vi "przygotowanie sygnalu do Mixed Graph.vi"() -> ()   [LabVIEW 2013]
uses:
  <vilib>/Waveform/DWDTOps.llb/DWDT Boolean Array to Digital.vi
panel:
  out "found":bool
  out "values":string
  out "transposed array":bool[][](array[boolean])
  in  "Array":bool[](array[boolean])
  out "Mixed Signal Graph":T1(graph)
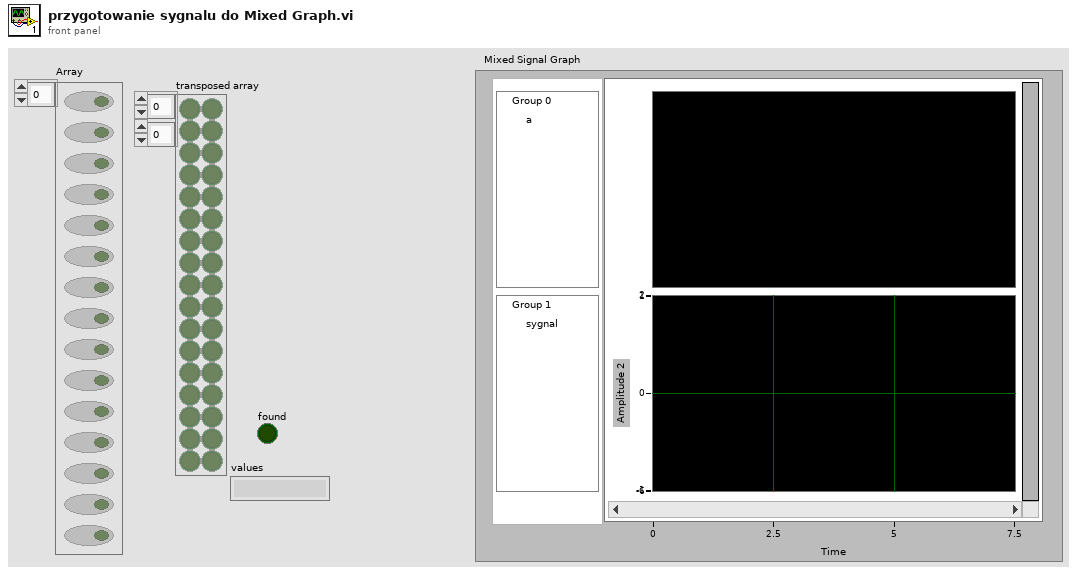
[diagram p1: front panel]
types:
  T1 = cluster{"digital waveform":digitalwaveform, waveform(dbl)}
  T2 = cluster{"digital waveform":digitalwaveform, "Waveform":waveform(dbl)}
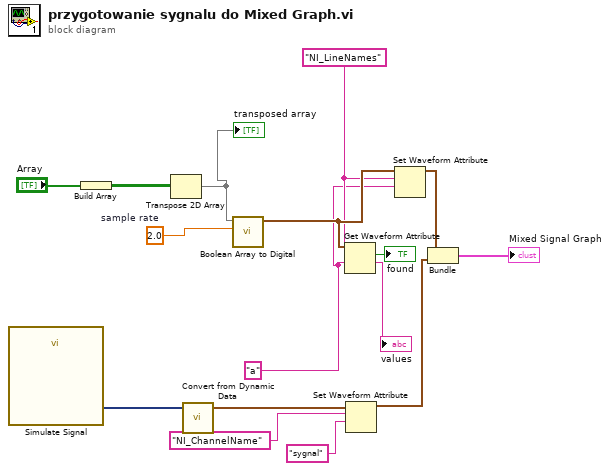
[diagram p0: block diagram]
diagram:
  w1 = "a" ("name")
  w3 = "NI_LineNames" ("name")
  w16 = 2.0  # sample rate
  n1 = call "Simulate Signal"() -> ("Sine"=w8:dynamicdata)  [unwired: 14 in, 1 out]
  n2 = Build Array("Array") -> (w14:bool[][])
  n3 = Transpose 2D Array(2D array=w14) -> (transposed array=w13:bool[][])
  "transposed array" <- w13
  n4 = call "Convert from Dynamic Data"("Dynamic Data Type"=w8) -> ("Waveform"=w7:waveform(dbl))  [unwired: 3 in]
  n5 = call-poly <vilib>:"Boolean Array to Digital.vi"("sample rate"=w16, "boolean array"=w13) -> ("digital waveform"=w4:digitalwaveform)  [unwired: 8 in, 1 out]
  n6 = Get Waveform Attribute(5:w1, 6:w3, 7:w4) -> (1:→"values":string, 2:→"found":bool)  [unwired: 1 in, 2 out]
  n7 = Set Waveform Attribute(5:"sygnal" ("name"), 6:"NI_ChannelName" ("name"), 7:w7) -> (3:w9:waveform(dbl))  [unwired: 1 in, 2 out]
  n8 = Set Waveform Attribute(5:w1, 6:w3, 7:w4) -> (3:w2:digitalwaveform)  [unwired: 1 in, 2 out]
  n9 = Bundle("digital waveform"=w2, "Waveform"=w9) -> (→"Mixed Signal Graph":T2)  [unwired: 1 in]
